vi "Configure Export Signal.vi"(8 "error in":errorcluster, 11 "Scope PXI CFG in":refnum<class "Scope PXI CFG.lvclass">) -> (0 "error out":errorcluster, 3 "Scope PXI CFG out":refnum<class "Scope PXI CFG.lvclass">)   [LabVIEW 2023, in "Scope.lvlib" / "Scope PXI.lvlib" / "Scope PXI CFG.lvclass"]
uses:
  Scope PXI CFG.lvclass
  <instrlib>/niScope/Controls/niScope exportable signals.ctl
  <instrlib>/niScope/Controls/niScope export destinations.ctl
  Scope PXI CFG.lvclass/Scope PXI CFG.ctl
  Configuration Base/Configuration Base.lvclass/Configuration Base.ctl
  c8bb0508-7956-418a-a24e-ae04bd9a5285.vi
  eeedd880-040e-4334-9e90-55d09acfd16d.vi
  2730e925-9606-4ad7-9a46-8b9e9f9d343d.vi
  <vilib>/JDP Science/JSONtext/Next JSON Value.vi
  <vilib>/JDP Science/JSONtext/String Subset.vi
  <vilib>/JDP Science/JSONtext/Parsing/Advance past next JSON Value (inlined COPY).vi
  <vilib>/JDP Science/JSONtext/Parsing/Advance past whitespace.vi
  <vilib>/JDP Science/JSONtext/Parsing/Advance past String.vi
  <vilib>/JDP Science/JSONtext/Parsing/Advance past Number.vi
  <vilib>/JDP Science/JSONtext/Parsing/Advance past Line Ending.vi
  <vilib>/JDP Science/JSONtext/Parsing/Parse Full Path or Item Name.vi
  <vilib>/JDP Science/JSONtext/Parsing/Advance past Array.vi
  <vilib>/JDP Science/JSONtext/Parsing/Advance past Object.vi
  <vilib>/JDP Science/JSONtext/support/Error Cluster From Code.vi
  <vilib>/JDP Science/JSONtext/Offset/Find Item Locations by Path.vi
  <vilib>/JDP Science/JSONtext/JSON text to Variant.vi
  <vilib>/Utility/error.llb/Error Cluster From Error Code.vi
  <vilib>/JDP Science/JSONtext/LVClass Serializer/JSONtext LVClass Serializer.lvclass
  <vilib>/ErrorRing/Error Ring.xnode
  Configuration Base/Configuration Base.lvclass
  <vilib>/JDP Science/JSONtext/JSONtext.lvlib
panel:
  out "signal":T1 caption="signal (Start Trigger)" items=["None"=0, "Start Trigger"=2, "Advance Trigger"=5, "Reference Trigger"=1, "End of Record Event"=4, "End of Acquisition Event"=3, "Ready for Start Event"=7, "Ready for Advance Event"=6, "Ready for Reference Event"=10, "Reference Clock"=100, "Sample Clock"=101, "5 Volt Power"=13]
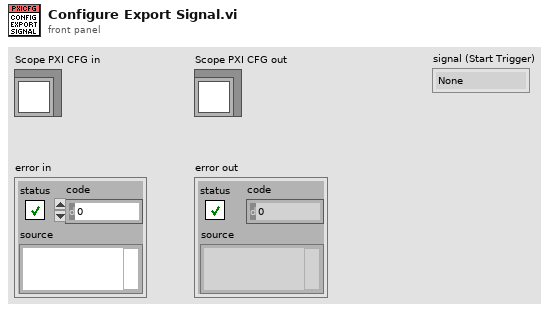
[diagram p1: front panel]
types:
  T1 = typedef "niScope exportable signals.ctl" = u16
  T2 = typedef "niScope export destinations.ctl" = string
  T3 = typedef "LVStringsAndValuesArrayTypeDef_U16.ctl" = cluster{"String":string, "Value":u16}[]
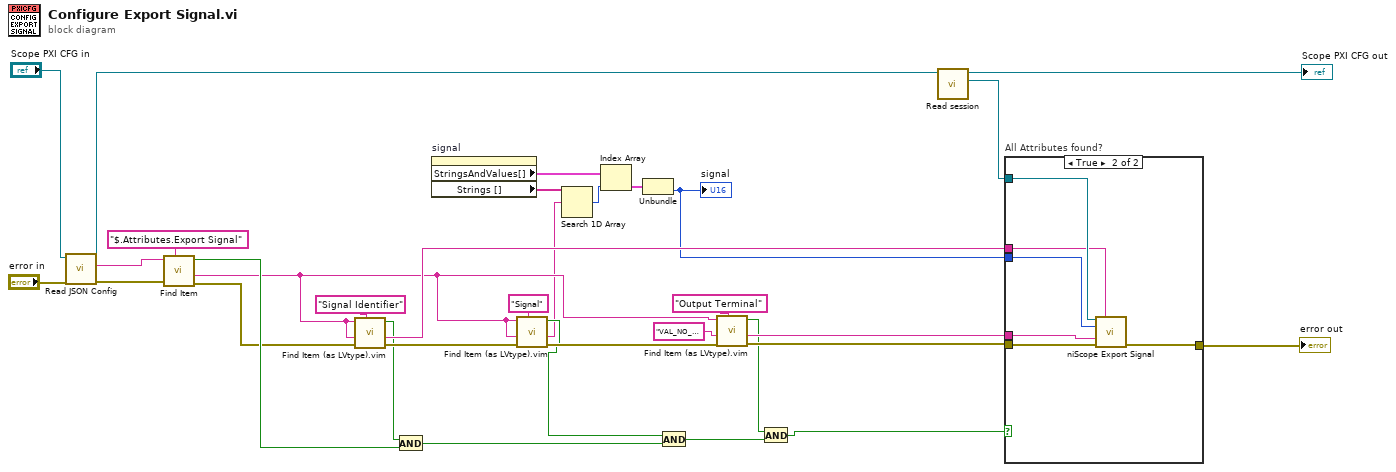
[diagram p0: block diagram]
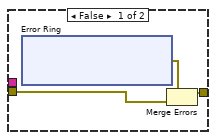
[diagram p2: hidden frame]
diagram:
  n1 = call "Read JSON Config.vi"("error in"="error in", "object in"="Scope PXI CFG in") -> ("error out"=w32:errorcluster, "<JSON>Config"=w29:string, "object out"=w30:refnum<class "Scope PXI CFG.lvclass">)  [unwired: 7 in]
  n2 = call <vilib>:"Find Item.vi"("$Path or Item Name"="$.Attributes.Export Signal", "error in (no error)"=w32, "JSON"=w29) -> ("error out"=w27:errorcluster, "<JSON>"=w7:string, "Found"=w28:bool)  [unwired: 5 in, 1 out]
  n3 = call "Find Item (as LVtype).vim"("$Path or Item Name"="Signal Identifier", "error in (no error)"=w27, "Data Type and Default Value"=w7, "JSON"=w7) -> ("error out"=w24:errorcluster, "Data"=w23:string, "Found"=w18:bool)  [unwired: 4 in, 1 out]
  n4 = And(x=w18, y=w28) -> (x .and. y?=w16:bool)
  n5 = property on="signal" class="Ring (strict)"() -> ("StringsAndValues[]"=w4:T3, "Strings []"=w6:string[])  [unwired: 2 in, 2 out]
  n6 = call "Find Item (as LVtype).vim"("$Path or Item Name"="Signal", "error in (no error)"=w24, "Data Type and Default Value"=w7, "JSON"=w7) -> ("error out"=w21:errorcluster, "Data"=w5:string, "Found"=w17:bool)  [unwired: 4 in, 1 out]
  n7 = Search 1D Array(1D array=w6, element=w5) -> (index of element=w3:i32)  [unwired: 1 in]
  n8 = Index Array(array=w4, index=w3) -> (element=w2:cluster{"String":string, "Value":u16})
  n9 = Unbundle(w2) -> ("Value"=w1:u16)  [unwired: 1 out]
  "signal" <- w1
  n10 = And(x=w17, y=w16) -> (x .and. y?=w14:bool)
  n11 = call "Find Item (as LVtype).vim"("$Path or Item Name"="Output Terminal", "error in (no error)"=w21, "Data Type and Default Value"=T2 "VAL_NO_SOURCE" ("output terminal"), "JSON"=w7) -> ("error out"=w20:errorcluster, "Data"=w19:T2, "Found"=w15:bool)  [unwired: 4 in, 1 out]
  n12 = And(x=w15, y=w14) -> (x .and. y?=w8:bool)
  n13 = call "Read session.vi"("Scope PXI CFG in"=w30) -> ("session"=w31:refnum<k15>, "Scope PXI CFG out"=→"Scope PXI CFG out":refnum<class "Scope PXI CFG.lvclass">)  [unwired: 8 in, 1 out]
  n14 = case "All Attributes found?" shown="True" w8 {
    tunnel: w20 -> [w34 w46]
    tunnel: w23 -> [_ w44]
    tunnel: w1 -> [_ w43]
    tunnel: [w35 w45] -> w11
    tunnel: w19 -> [_ w42]
    tunnel: w31 -> [_ w47]
    frame False {
      n15 = xnode "Error Ring"() -> ("error out"=w36:errorcluster)
      n16 = Merge Errors(w36, w34) -> (w35:errorcluster)
    }
    frame True {
      n17 = call <instrlib>:"niScope Export Signal.vi"("instrument handle"=w47, "signal identifier"=w44, "signal"=w43, "output terminal"=w42, "error in"=w46) -> ("error out"=w45:errorcluster)  [unwired: 9 in, 1 out]
    }
  }
  "error out" <- w11
